vi "PAN_MacroChange.vi"(8 "error in (no error)":errorcluster, 9 "action":enum16{"add", "delete"}(ring), 10 "argument":string) -> (0 "error out":errorcluster)   [LabVIEW 2016]
uses:
  <vilib>/Utility/error.llb/DialogType.ctl
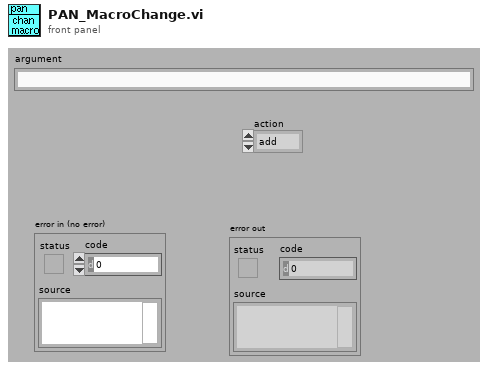
[diagram p1: front panel]
types:
  T1 = typedef "DialogType.ctl" = u16
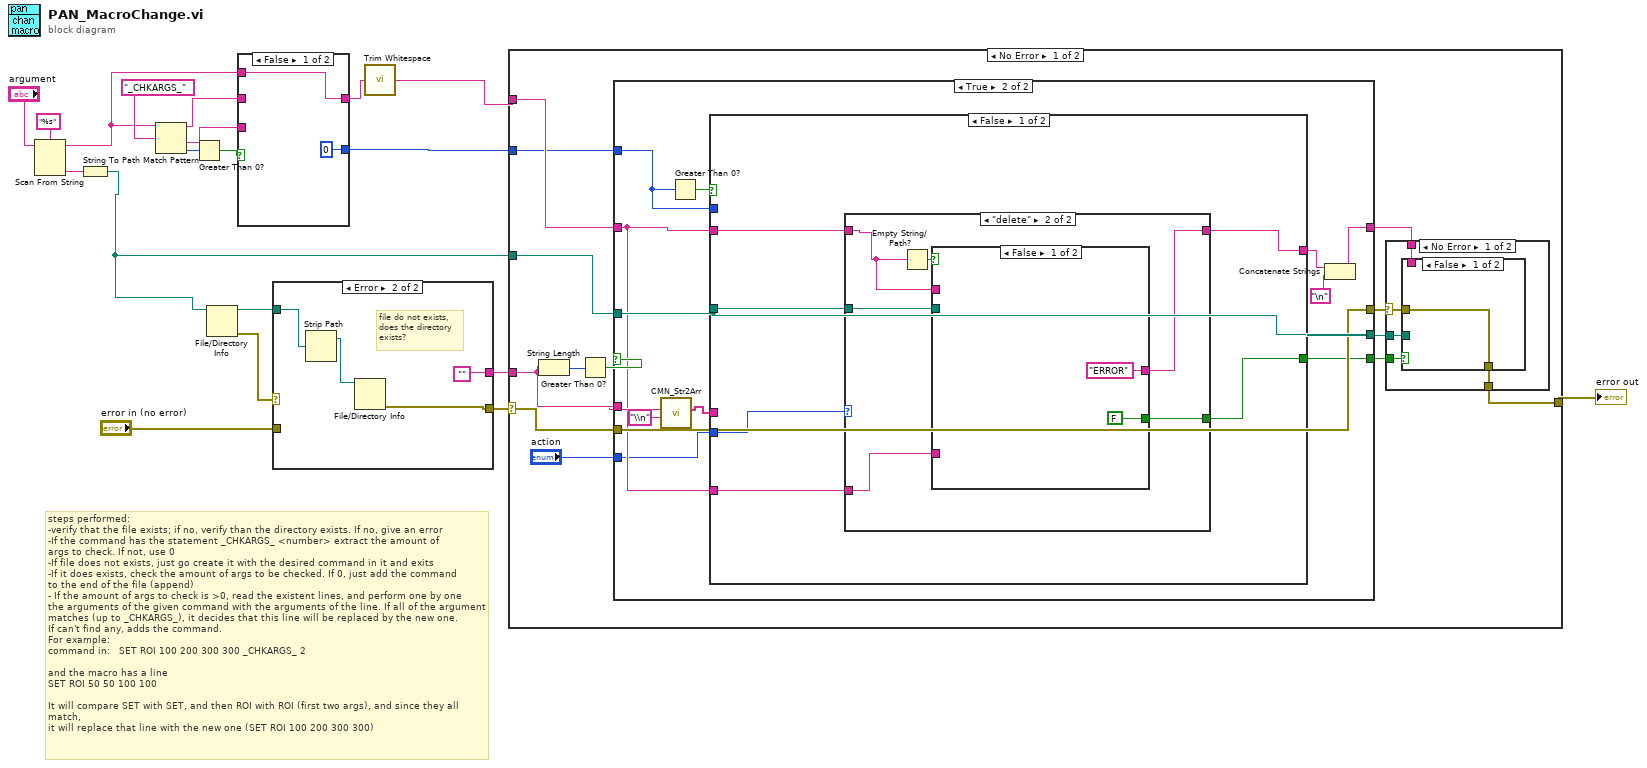
[diagram p0: block diagram]
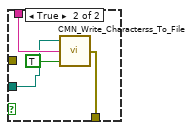
[diagram p2: hidden frame]
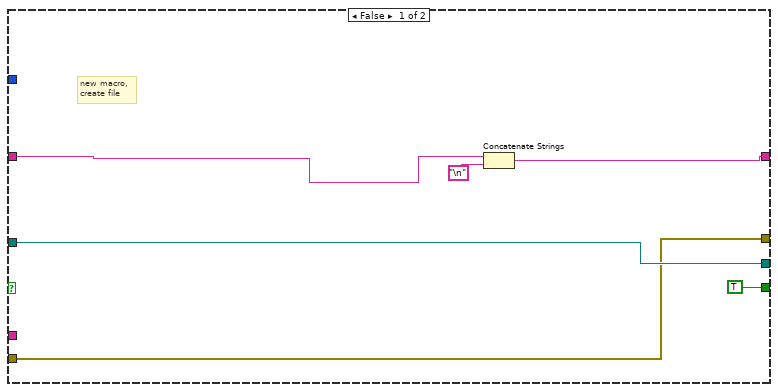
[diagram p4: hidden frame]
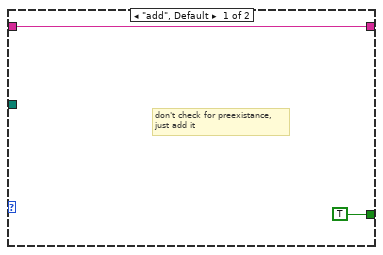
[diagram p5: hidden frame]
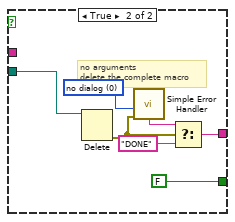
[diagram p6: hidden frame]
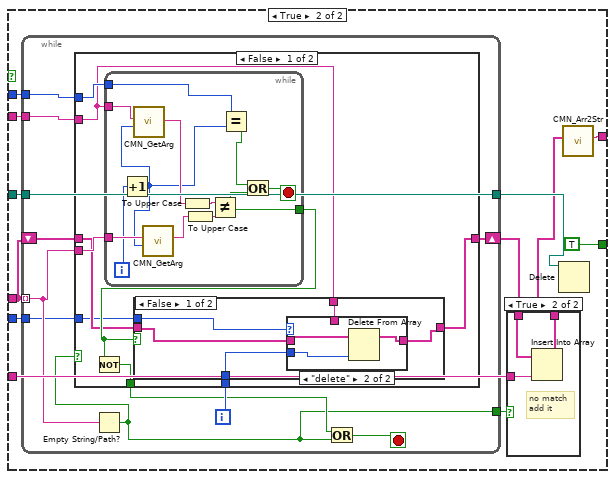
[diagram p7: hidden frame]
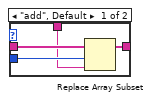
[diagram p9: hidden frame]
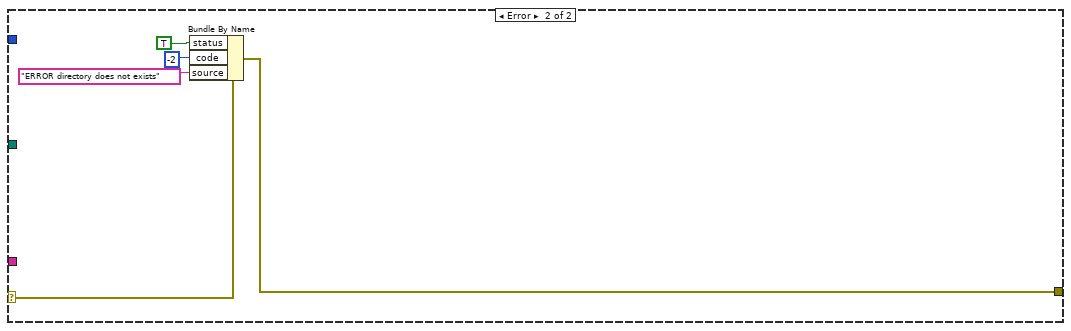
[diagram p12: hidden frame]
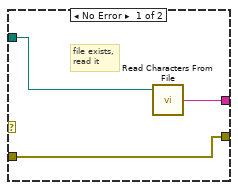
[diagram p13: hidden frame]
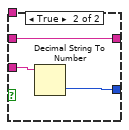
[diagram p14: hidden frame]
diagram:
  # "steps performed:\n-verify that the file exists; if no, verify than the directory exists. If no, give an error\n-If the command has the statement _CHKARGS_ <number> extract the amount of\nargs to check. If not, use 0\n-If file does not exists, just go create it with the desired command in it and exits\n-If it does exists, check the amount of args to be checked. If 0, just add the command\nto the end of the file (append)\n- If the amount of args to check is >0, read the existent lines, and perform one by one\nthe arguments of the given command with the arguments of the line. If all of the argument\nmatches (up to _CHKARGS_), it decides that this line will be replaced by the new one.\nIf can't find any, adds the command. \nFor example:\ncommand in:   SET ROI 100 200 300 300 _CHKARGS_ 2\n\nand the macro has a line\nSET ROI 50 50 100 100\n\nIt will compare SET with SET, and then ROI with ROI (first two args), and since they all match,\nit will replace that line with the new one (SET ROI 100 200 300 300)"
  n1 = Scan From String(format string="%s", input string="argument") -> (remaining string=w11:string, output 1=w17:string)  [unwired: 2 in, 3 out]
  n2 = String To Path(string=w17) -> (path=w4:path)
  n3 = Match Pattern(string=w11, regular expression="_CHKARGS_") -> (before substring=w12:string, after substring=w13:string, offset past match=w15:i32)  [unwired: 2 out]
  n4 = Greater Than 0?(x=w15) -> (x > 0?=w14:bool)
  n5 = File/Directory Info(path=w4) -> (path out=w8:path, error out=w10:errorcluster)  [unwired: 1 in, 5 out]
  n6 = case shown="False" w14 {
    tunnel: w13 -> [_ w24]
    tunnel: [0 w23] -> w5
    tunnel: w12 -> [_ w22]
    tunnel: [w20 w22] -> w2
    tunnel: w11 -> [w20 _]
    frame False {
    }
    frame True {
      n7 = Decimal String To Number(string=w24) -> (number=w23:i32)  [unwired: 3 out]
    }
  }
  n8 = case shown="Error" w10 {
    tunnel: "error in (no error)" -> [w26 _]
    tunnel: w8 -> [w27 w31]
    tunnel: [w26 w29] -> w7
    tunnel: [w25 ""] -> w6
    frame No Error {
      # "file exists,\nread it"
      n9 = call <vilib>:"Read Characters From File.vi"("file path (dialog if empty)"=w27) -> ("character string"=w25:string)  [unwired: 1 in, 7 out]
    }
    frame Error {
      # "file do not exists,\ndoes the directory\nexists?"
      n10 = Strip Path(path=w31) -> (stripped path=w30:path)  [unwired: 1 out]
      n11 = File/Directory Info(path=w30) -> (error out=w29:errorcluster)  [unwired: 1 in, 6 out]
    }
  }
  n12 = call <vilib>:"Trim Whitespace.vi"("string"=w2) -> ("trimmed string"=w1:string)  [unwired: 1 in]
  n13 = case shown="No Error" w7 {
    selector: w7 -> [w36 w165]
    tunnel: w6 -> [w40 _]
    tunnel: w1 -> [w42 _]
    tunnel: w5 -> [w39 _]
    tunnel: w4 -> [w41 _]
    tunnel: [w34 w161] -> w3
    frame No Error {
      n14 = String Length(string=w40) -> (length=w44:i32)
      n15 = Greater Than 0?(x=w44) -> (x > 0?=w43:bool)
      n16 = case shown="True" w43 {
        tunnel: w42 -> [w59 w67]
        tunnel: w41 -> [w61 w68]
        tunnel: w40 -> [_ w73]
        tunnel: w39 -> [_ w70]
        tunnel: [w61 w68] -> w38
        tunnel: [w57 w64] -> w37
        tunnel: [w60 w71] -> w35
        tunnel: w36 -> [w60 w71]
        tunnel: "action" -> [_ w63]
        tunnel: [TRUE ("append to file? (new file:F)") w62] -> w32
        frame False {
          # "new macro,\ncreate file"
          n17 = Concatenate Strings(w59, "\n") -> (w57:string)
        }
        frame True {
          n18 = call "CMN_Str2Arr.vi"("separator"="\\n", "string in"=w73) -> ("Array out"=w72:string[])  [unwired: 2 in, 7 out]
          n19 = Greater Than 0?(x=w70) -> (x > 0?=w69:bool)
          n20 = case shown="False" w69 {
            tunnel: w67 -> [w79 w109]
            tunnel: w70 -> [_ w108]
            tunnel: w72 -> [_ w106]
            tunnel: [w78 w107] -> w66
            tunnel: w68 -> [w77 w105]
            tunnel: w67 -> [w76 w100]
            tunnel: w63 -> [w80 w99]
            tunnel: [w75 TRUE ("append to file? (new file:F)")] -> w62
            frame False {
              n21 = case shown="\"delete\"" w80 {
                tunnel: w79 -> [w82 w85]
                tunnel: [w82 w86] -> w78
                tunnel: w77 -> [_ w87]
                tunnel: w76 -> [_ w84]
                tunnel: [TRUE ("append to file? (new file:F)") w83] -> w75
                frame "add", Default {
                  # "don't check for preexistance,\njust add it"
                }
                frame "delete" {
                  n22 = Empty String/Path?(string/path=w85) -> (empty?=w88:bool)
                  n23 = case shown="False" w88 {
                    tunnel: w87 -> [_ w97]
                    tunnel: ["ERROR" ("f") w92] -> w86
                    tunnel: w85 -> [_ _]
                    tunnel: w84 -> [_ _]
                    tunnel: [FALSE ("append to file? (new file:F)") FALSE ("append to file? (new file:F)")] -> w83
                    frame False {
                    }
                    frame True {
                      w95 = T1 0 items=["no dialog", "OK message", "continue or stop message", "OK message + warnings", "continue/stop + warnings"] ("type of dialog (OK msg:1)")
                      # "no arguments\ndelete the complete macro"
                      n24 = Delete(path (use dialog)=w97) -> (error out=w96:errorcluster)  [unwired: 1 in, 5 out]
                      n25 = call <vilib>:"Simple Error Handler.vi"("type of dialog (OK msg:1)"=w95, "error in (no error)"=w96) -> ("message"=w94:string)  [unwired: 7 out]
                      n26 = Select(t=w94, s=w96, f="DONE") -> (s? t:f=w92:string)
                    }
                  }
                }
              }
            }
            frame True {
              n27 = while {
                tunnel: w106 -> [w122] mode=indexing
                tunnel: w109 -> [w124]
                tunnel: w108 -> [w123]
                shift-right: [w119] -> w102
                shift-left: w106 -> [w120]
                tunnel: w105 -> [w116]
                tunnel: [w116] -> w104
                tunnel: [w115] -> w103
                tunnel: w99 -> [w114]
                i -> [w118]
                stop <- w121 stop-if-true
                n28 = Empty String/Path?(string/path=w122) -> (empty?=w115:bool)
                n29 = case shown="False" w115 {
                  selector: w115 -> [_ w159]
                  tunnel: w124 -> [w126 _]
                  tunnel: w123 -> [w133 _]
                  tunnel: w122 -> [w132 _]
                  tunnel: [w130 w159] -> w117
                  tunnel: w120 -> [w129 w160]
                  tunnel: [w128 w160] -> w119
                  tunnel: w118 -> [w127 _]
                  tunnel: w114 -> [w125 _]
                  frame False {
                    n30 = while {
                      tunnel: w132 -> [w158]
                      tunnel: w126 -> [w157]
                      tunnel: w133 -> [w152]
                      tunnel: [w153] -> w131
                      i -> [w150]
                      stop <- w154 stop-if-true
                      n31 = Increment(x=w150) -> (x+1=w149:i32)
                      n32 = call "CMN_GetArg.vi"("arg number"=w149, "arguments"=w157) -> ("argument"=w155:string)  [unwired: 9 out]
                      n33 = call "CMN_GetArg.vi"("arg number"=w149, "arguments"=w158) -> ("argument"=w156:string)  [unwired: 9 out]
                      n34 = To Upper Case(1:w155) -> (0:w148:string)
                      n35 = To Upper Case(1:w156) -> (0:w147:string)
                      n36 = Not Equal?(x=w148, y=w147) -> (x != y?=w153:bool)
                      n37 = Equal?(x=w152, y=w149) -> (x = y?=w151:bool)
                      n38 = Or(x=w151, y=w153) -> (x .or. y?=w154:bool)
                    }
                    n39 = Not(x=w131) -> (.not. x?=w130:bool)
                    n40 = case shown="False" w131 {
                      tunnel: w129 -> [w138 w146]
                      tunnel: [w135 w146] -> w128
                      tunnel: w127 -> [w137 _]
                      tunnel: w126 -> [w136 _]
                      tunnel: w125 -> [w134 _]
                      frame False {
                        n41 = case shown="\"delete\"" w134 {
                          tunnel: w138 -> [w142 w145]
                          tunnel: w137 -> [w141 w143]
                          tunnel: w136 -> [w140 _]
                          tunnel: [w139 w144] -> w135
                          frame "add", Default {
                            n42 = Replace Array Subset(array=w142, new element=w140, index=w141) -> (w139:string[])
                          }
                          frame "delete" {
                            n43 = Delete From Array(array=w145, index=w143) -> (array with subset deleted=w144:string[])  [unwired: 1 in, 1 out]
                          }
                        }
                      }
                      frame True {
                      }
                    }
                  }
                  frame True {
                  }
                }
                n44 = Or(x=w117, y=w115) -> (x .or. y?=w121:bool)
              }
              n45 = case shown="True" w103 {
                tunnel: w102 -> [w110 w113]
                tunnel: [w110 w112] -> w101
                tunnel: w100 -> [_ w111]
                frame False {
                }
                frame True {
                  # "no match\nadd it"
                  n46 = Insert Into Array(array=w113, new element=w111) -> (w112:string[])  [unwired: 1 in]
                }
              }
              n47 = Delete(path (use dialog)=w104) -> ()  [unwired: 1 in, 6 out]
              n48 = call "CMN_Arr2Str.vi"("Array in"=w101) -> ("string out"=w107:string)  [unwired: 10 out]
            }
          }
          n49 = Concatenate Strings(w66, "\n") -> (w64:string)
        }
      }
      n50 = case shown="No Error" w35 {
        selector: w35 -> [w45 w55]
        tunnel: w38 -> [w47 _]
        tunnel: w37 -> [w49 _]
        tunnel: [w48 w55] -> w34
        tunnel: w32 -> [w46 _]
        frame No Error {
          n51 = case shown="False" w46 {
            tunnel: w49 -> [_ w54]
            tunnel: [w50 w53] -> w48
            tunnel: w47 -> [_ w52]
            tunnel: w45 -> [w50 _]
            frame False {
            }
            frame True {
              n52 = call "CMN_Write_Characterss_To_File.vi"("append to file? (new file:F)"=TRUE, "character string"=w54, "file path (dialog if empty)"=w52) -> ("error out"=w53:errorcluster)  [unwired: 2 out]
            }
          }
        }
        frame Error {
        }
      }
    }
    frame Error {
      n53 = Bundle By Name(cluster=w165, "status"=TRUE, "code"=-2, "source"="ERROR directory does not exists") -> (w161:errorcluster)
    }
  }
  "error out" <- w3
